vi "set_in_library.vi"(2 "Cluster":T4, 3 "camera cluster":T3, 4 "Tracker Handle":i32, 5 "Array":dbl[][](array[numeric])) -> (0 "No Error":bool, 1 "Directory Exists?":bool)   [LabVIEW 2010]
uses:
  <vilib>/vision/Avi1.llb/AviRefnum.ctl
  <vilib>/userDefined/High Color/IMAQdx.ctl
  lib/MWT.dll
panel:
  out "return type 9":i32
  out "return type 8":i32
  out "return type 7":i32
  out "return type 6":i32
  out "return type 5":i32
  out "return type 4":i32
  out "return type 3":i32
  out "return type 2":i32
  out "return type":i32
  in  "ObjectFrames of Persistence":i32=5
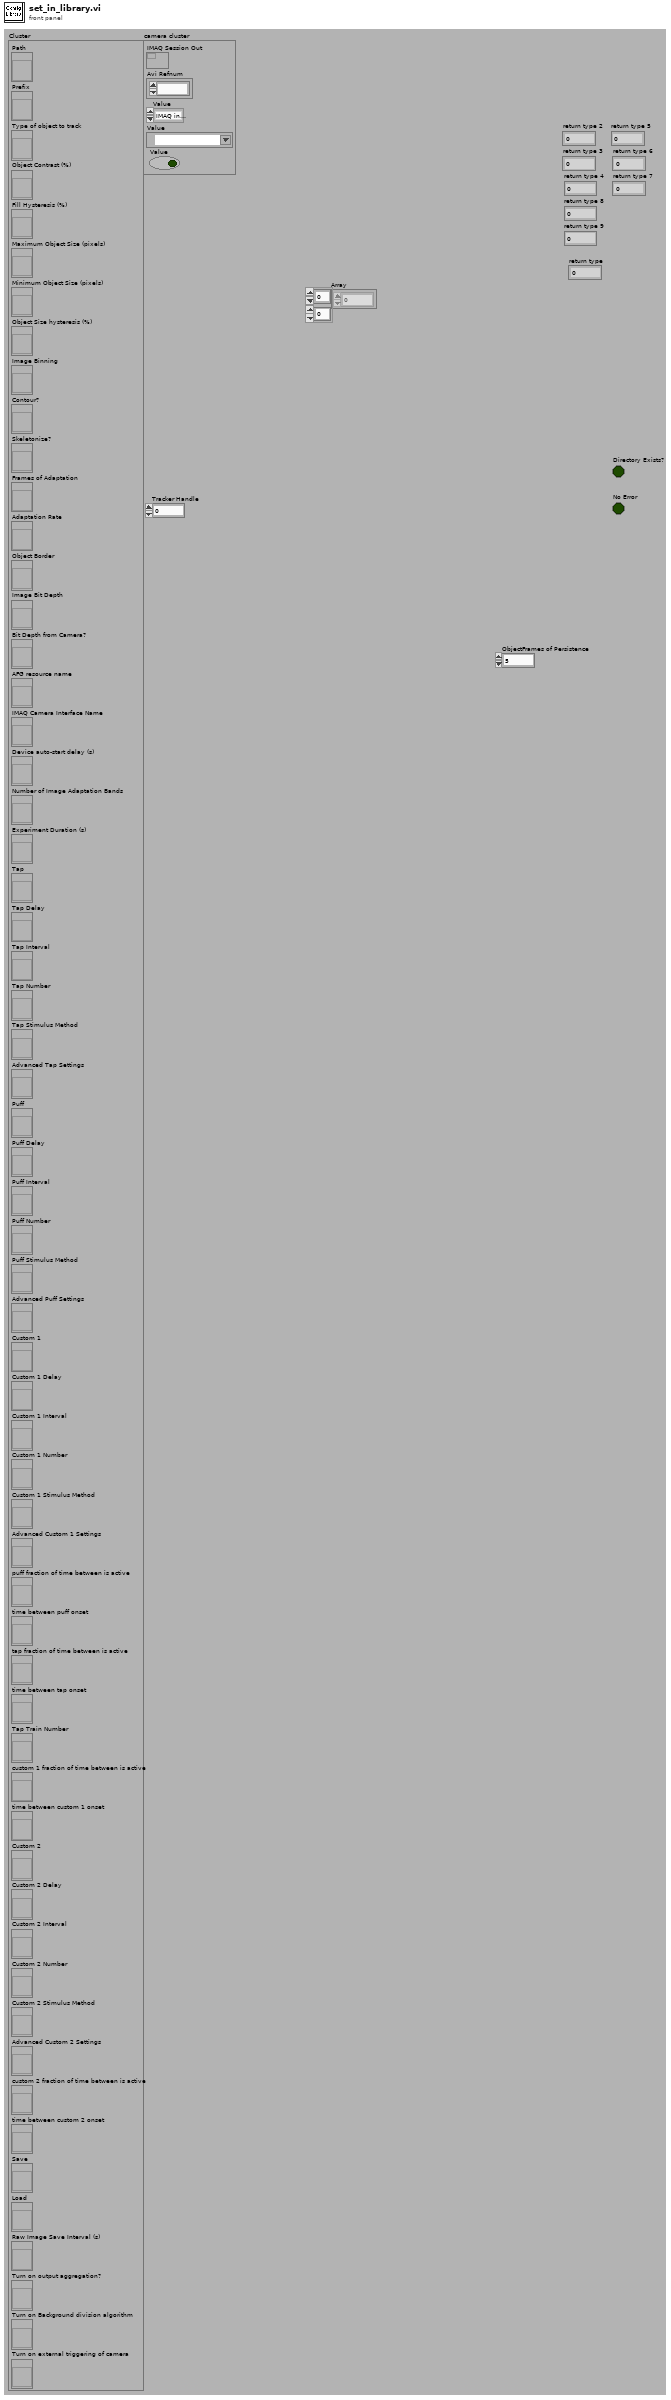
[diagram p1: front panel]
types:
  T1 = typedef "AviRefnum.ctl" = refnum<k1>
  T2 = typedef "IMAQdx.ctl" = refnum<k21>
  T3 = cluster{"IMAQ Session Out":refnum<k11>, "Avi Refnum":T1, "Value":enum32{"IMAQ interface", "IMAQdx interface", "AVI file"}, "Value":T2, "Value":bool}
  T4 = cluster{"Path":refnum<vi>, "Prefix":refnum<vi>, "Type of object to track":refnum<vi>, "Object Contrast (%)":refnum<vi>, "Fill Hysteresis (%)":refnum<vi>, "Maximum Object Size (pixels)":refnum<vi>, "Minimum Object Size (pixels)":refnum<vi>, "Object Size hysteresis (%)":refnum<vi>, "Image Binning":refnum<vi>, "Contour?":refnum<vi>, "Skeletonize?":refnum<vi>, "Frames of Adaptation":refnum<vi>, "Adaptation Rate":refnum<vi>, "Object Border":refnum<vi>, "Image Bit Depth":refnum<vi>, "Bit Depth from Camera?":refnum<vi>, "AFG resource name":refnum<vi>, "IMAQ Camera Interface Name":refnum<vi>, "Device auto-start delay (s)":refnum<vi>, "Number of Image Adaptation Bands":refnum<vi>, "Experiment Duration (s)":refnum<vi>, "Tap":refnum<vi>, "Tap Delay":refnum<vi>, "Tap Interval":refnum<vi>, "Tap Number":refnum<vi>, "Tap Stimulus Method":refnum<vi>, "Advanced Tap Settings":refnum<vi>, "Puff":refnum<vi>, "Puff Delay":refnum<vi>, "Puff Interval":refnum<vi>, "Puff Number":refnum<vi>, "Puff Stimulus Method":refnum<vi>, "Advanced Puff Settings":refnum<vi>, "Custom 1":refnum<vi>, "Custom 1 Delay":refnum<vi>, "Custom 1 Interval":refnum<vi>, "Custom 1 Number":refnum<vi>, "Custom 1 Stimulus Method":refnum<vi>, "Advanced Custom 1 Settings":refnum<vi>, "puff fraction of time between is active":refnum<vi>, "time between puff onset":refnum<vi>, "tap fraction of time between is active":refnum<vi>, "time between tap onset":refnum<vi>, "Tap Train Number":refnum<vi>, "custom 1 fraction of time between is active":refnum<vi>, "time between custom 1 onset":refnum<vi>, "Custom 2":refnum<vi>, "Custom 2 Delay":refnum<vi>, "Custom 2 Interval":refnum<vi>, "Custom 2 Number":refnum<vi>, "Custom 2 Stimulus Method":refnum<vi>, "Advanced Custom 2 Settings":refnum<vi>, "custom 2 fraction of time between is active":refnum<vi>, "time between custom 2 onset":refnum<vi>, "Save":refnum<vi>, "Load":refnum<vi>, "Raw Image Save Interval (s)":refnum<vi>, "Turn on output aggregation?":refnum<vi>, "Turn on Background division algorithm":refnum<vi>, "Turn on external triggering of camera":refnum<vi>}
  T5 = cluster{"Value":path, "Value":string, "Value":bool, "Value":dbl, "Value":dbl, "Value":i32, "Value":i32, "Value":dbl, "Value":u16, "Value":bool, "Value":bool, "Value":i32, "Value":i32, "Value":i32, "Value":u32, "Value":i32, "Value":bool}
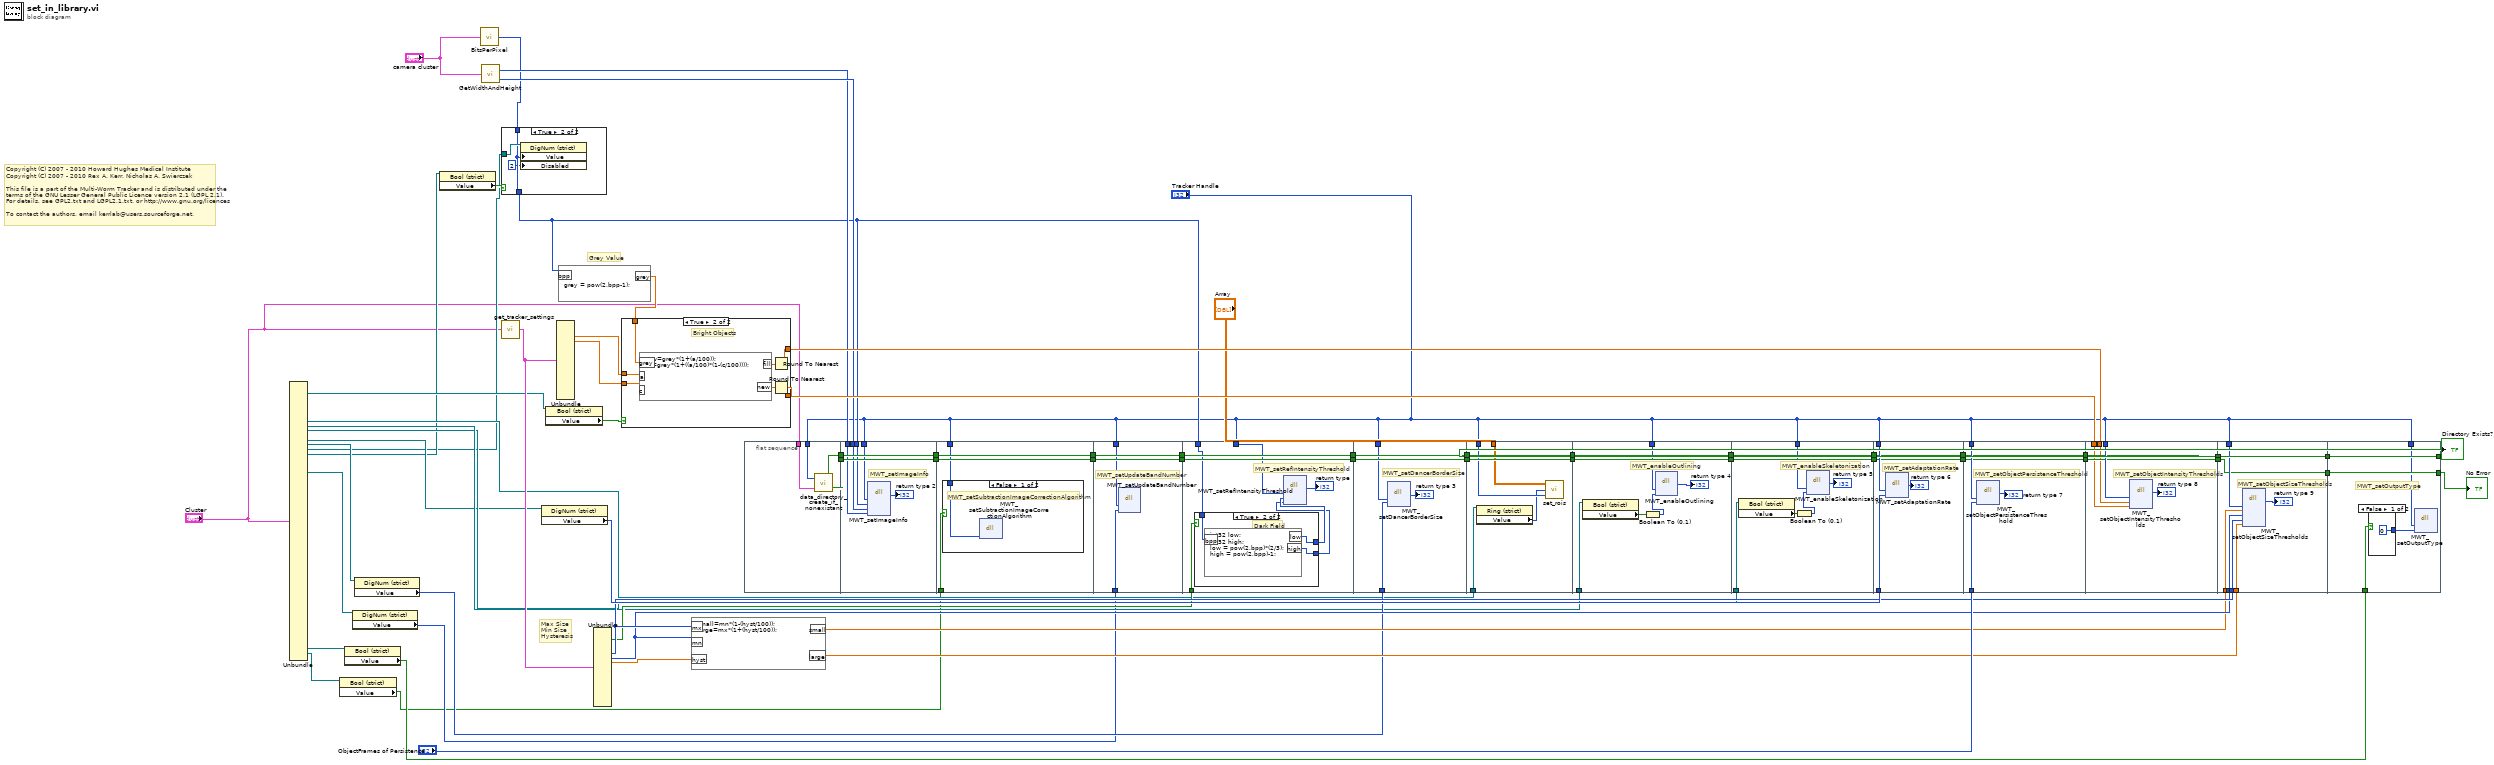
[diagram p0: block diagram]
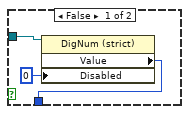
[diagram p2: hidden frame]
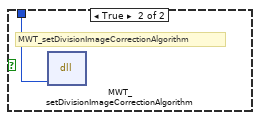
[diagram p3: hidden frame]
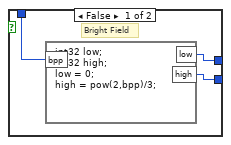
[diagram p4: hidden frame]
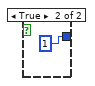
[diagram p5: hidden frame]
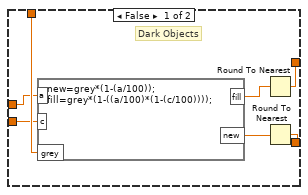
[diagram p6: hidden frame]
diagram:
  # "Copyright (C) 2007 - 2010 Howard Hughes Medical Institute\nCopyright (C) 2007 - 2010 Rex A. Kerr, Nicholas A. Swierczek\n \nThis file is a part of the Multi-Worm Tracker and is distributed under the\nterms of the GNU Lesser General Public Licence version 2.1 (LGPL 2.1).\nFor details, see GPL2.txt and LGPL2.1.txt, or http://www.gnu.org/licences\n \nTo contact the authors, email kerrlab@users.sourceforge.net."
  # "Max Size\nMin Size\nHysteresis"
  # "Grey Value"
  n1 = Unbundle("Cluster") -> ("Type of object to track"=w25:refnum<vi>, "Image Binning"=w24:refnum<vi>, "Contour?"=w23:refnum<vi>, "Skeletonize?"=w22:refnum<vi>, "Adaptation Rate"=w21:refnum<vi>, "Object Border"=w20:refnum<vi>, "Image Bit Depth"=w18:refnum<vi>, "Bit Depth from Camera?"=w19:refnum<vi>, "Number of Image Adaptation Bands"=w15:refnum<vi>, "Turn on output aggregation?"=w11:refnum<vi>, "Turn on Background division algorithm"=w5:refnum<vi>)  [unwired: 49 out]
  n2 = property class="Bool (strict)"(reference=w5) -> ("Value"=w4:bool)  [unwired: 1 in, 2 out]
  n3 = property class="Bool (strict)"(reference=w11) -> ("Value"=w10:bool)  [unwired: 1 in, 2 out]
  n4 = property class="DigNum (strict)"(reference=w15) -> ("Value"=w14:i32)  [unwired: 1 in, 2 out]
  n5 = property class="DigNum (strict)"(reference=w20) -> ("Value"=w31:i32)  [unwired: 1 in, 2 out]
  n6 = property class="Bool (strict)"(reference=w19) -> ("Value"=w42:bool)  [unwired: 1 in, 2 out]
  n7 = call "BitsPerPixel.vi"("camera cluster"="camera cluster") -> ("BitsPerPixel"=w28:u32)
  n8 = call "GetWidthAndHeight.vi"("camera cluster"="camera cluster") -> ("Width"=w29:u32, "Height"=w30:u32)
  n9 = call "get_tracker_settings.vi"("Cluster"="Cluster") -> ("settings value cluster"=w66:T5)
  n10 = case shown="True" w42 {
    tunnel: [w69 w72] -> w27
    tunnel: w28 -> [_ w72]
    tunnel: w18 -> [w70 w73]
    frame False {
      n11 = property class="DigNum (strict)"(reference=w70, "Disabled"=u8 0) -> ("Value"=w69:u32)  [unwired: 1 in, 2 out]
    }
    frame True {
      n12 = property class="DigNum (strict)"(reference=w73, "Value"=w72, "Disabled"=u8 2) -> ()  [unwired: 1 in, 2 out]
    }
  }
  n13 = property class="DigNum (strict)"(reference=w21) -> ("Value"=w62:i32)  [unwired: 1 in, 2 out]
  n14 = property class="Bool (strict)"(reference=w25) -> ("Value"=w67:bool)  [unwired: 1 in, 2 out]
  n15 = Unbundle(w66) -> ("Value"=w37:dbl, "Value"=w65:dbl)  [unwired: 15 out]
  n16 = formula code="grey = pow(2,bpp-1);"("bpp"=w27) -> ("grey"=w43:dbl)
  n17 = Unbundle(w66) -> ("Value"=w26:bool, "Value"=w36:i32, "Value"=w35:i32, "Value"=w34:dbl)  [unwired: 13 out]
  n18 = case shown="True" w67 {
    tunnel: w43 -> [w80 w87]
    tunnel: w37 -> [w79 w86]
    tunnel: w65 -> [w78 w85]
    tunnel: [w74 w81] -> w64
    tunnel: [w76 w83] -> w63
    frame False {
      # "Dark Objects"
      n19 = formula code="new=grey*(1-(a/100));\nfill=grey*(1-((a/100)*(1-(c/100))));"("a"=w79, "c"=w78, "grey"=w80) -> ("new"=w77:dbl, "fill"=w75:dbl)
      n20 = Round To Nearest(number=w75) -> (nearest integer value=w74:dbl)
      n21 = Round To Nearest(number=w77) -> (nearest integer value=w76:dbl)
    }
    frame True {
      # "Bright Objects"
      n22 = formula code="new=grey*(1+(a/100));\nfill=grey*(1+((a/100)*(1-(c/100))));"("a"=w86, "c"=w85, "grey"=w87) -> ("new"=w84:dbl, "fill"=w82:dbl)
      n23 = Round To Nearest(number=w82) -> (nearest integer value=w81:dbl)
      n24 = Round To Nearest(number=w84) -> (nearest integer value=w83:dbl)
    }
  }
  n25 = formula code="small=mn*(1-(hyst/100));\nlarge=mx*(1+(hyst/100));"("mx"=w36, "mn"=w35, "hyst"=w34) -> ("small"=w33:dbl, "large"=w32:dbl)
  n26 = flat-sequence {
    tunnel: [w91] -> w45
    tunnel: [w90] -> w44
    tunnel: "Tracker Handle" -> [w89]
    tunnel: "Cluster" -> [w88]
    tunnel: w45 -> [w98]
    tunnel: [w98] -> w9
    tunnel: w44 -> [w97]
    tunnel: [w97] -> w7
    tunnel: "Tracker Handle" -> [w96]
    tunnel: w27 -> [w95]
    tunnel: w29 -> [w94]
    tunnel: w30 -> [w93]
    tunnel: w9 -> [w102]
    tunnel: [w102] -> w8
    tunnel: w7 -> [w101]
    tunnel: [w101] -> w6
    tunnel: w4 -> [w100]
    tunnel: "Tracker Handle" -> [w99]
    tunnel: w8 -> [w108]
    tunnel: [w108] -> w17
    tunnel: w6 -> [w107]
    tunnel: [w107] -> w16
    tunnel: "Tracker Handle" -> [w106]
    tunnel: w14 -> [w105]
    tunnel: w17 -> [w116]
    tunnel: [w116] -> w49
    tunnel: w16 -> [w115]
    tunnel: [w115] -> w47
    tunnel: "Tracker Handle" -> [w114]
    tunnel: w27 -> [w111]
    tunnel: w26 -> [w112]
    tunnel: w49 -> [w127]
    tunnel: [w127] -> w48
    tunnel: w47 -> [w126]
    tunnel: [w126] -> w46
    tunnel: "Tracker Handle" -> [w125]
    tunnel: w31 -> [w124]
    tunnel: w48 -> [w133]
    tunnel: [w133] -> w41
    tunnel: w46 -> [w132]
    tunnel: [w132] -> w39
    tunnel: "Array" -> [w131]
    tunnel: "Tracker Handle" -> [w130]
    tunnel: w24 -> [w129]
    tunnel: w41 -> [w140]
    tunnel: [w140] -> w40
    tunnel: w39 -> [w139]
    tunnel: [w139] -> w38
    tunnel: "Tracker Handle" -> [w136]
    tunnel: w23 -> [w135]
    tunnel: [w147] -> w57
    tunnel: w40 -> [w147]
    tunnel: w38 -> [w146]
    tunnel: [w146] -> w56
    tunnel: "Tracker Handle" -> [w145]
    tunnel: w22 -> [w144]
    tunnel: w62 -> [w152]
    tunnel: "Tracker Handle" -> [w151]
    tunnel: [w150] -> w58
    tunnel: w57 -> [w150]
    tunnel: w56 -> [w149]
    tunnel: [w149] -> w55
    tunnel: "ObjectFrames of Persistence" -> [w157]
    tunnel: "Tracker Handle" -> [w156]
    tunnel: [w155] -> w59
    tunnel: w58 -> [w155]
    tunnel: w55 -> [w154]
    tunnel: [w154] -> w54
    tunnel: w64 -> [w159]
    tunnel: w63 -> [w160]
    tunnel: "Tracker Handle" -> [w163]
    tunnel: [w162] -> w60
    tunnel: w59 -> [w162]
    tunnel: w54 -> [w161]
    tunnel: [w161] -> w53
    tunnel: w33 -> [w171]
    tunnel: w35 -> [w170]
    tunnel: w36 -> [w169]
    tunnel: w32 -> [w168]
    tunnel: "Tracker Handle" -> [w167]
    tunnel: w60 -> [w166]
    tunnel: w53 -> [w165]
    tunnel: [w166] -> w13
    tunnel: [w165] -> w12
    tunnel: [w175] -> w51
    tunnel: [w176] -> w52
    tunnel: w13 -> [w176]
    tunnel: w12 -> [w175]
    tunnel: "Tracker Handle" -> [w173]
    tunnel: w10 -> [w172]
    frame #0 {
      n27 = call "data_directory_create_if_nonexistant.vi"("Cluster"=w88, "Tracker Handle"=w89) -> ("Error"=w90:bool, "Directory Exists?"=w91:bool)
    }
    frame #1 {
      # "MWT_setImageInfo"
      n28 = dll-call lib="C:/MWT/lib/MWT.dll" fn="MWT_setImageInfo"("handle"=w96, "bits"=w95, "width"=w93, "height"=w94) -> ("return type"=→"return type 2":i32)  [unwired: 7 in, 2 out]
    }
    frame #2 {
      n29 = case shown="False" w100 {
        tunnel: w99 -> [w103 w104]
        frame False {
          # "MWT_setSubtractionImageCorrectionAlgorithm"
          n30 = dll-call lib="C:/MWT/lib/MWT.dll" fn="MWT_setSubtractionImageCorrectionAlgorithm"("handle"=w103) -> ()  [unwired: 5 in, 2 out]
        }
        frame True {
          # "MWT_setDivisionImageCorrectionAlgorithm"
          n31 = dll-call lib="C:/MWT/lib/MWT.dll" fn="MWT_setDivisionImageCorrectionAlgorithm"("handle"=w104) -> ()  [unwired: 5 in, 2 out]
        }
      }
    }
    frame #3 {
      # "MWT_setUpdateBandNumber"
      n32 = dll-call lib="C:/MWT/lib/MWT.dll" fn="MWT_setUpdateBandNumber"("handle"=w106, "num_bands"=w105) -> ()  [unwired: 6 in, 2 out]
    }
    frame #4 {
      # "MWT_setRefIntensityThreshold"
      n33 = case shown="True" w112 {
        tunnel: [w119 w122] -> w110
        tunnel: [w118 w121] -> w109
        tunnel: w111 -> [w117 w120]
        frame False {
          # "Bright Field"
          n34 = formula code="int32 low;\nint32 high;\nlow = 0;\nhigh = pow(2,bpp)/3;"("bpp"=w117) -> ("low"=w119:i32, "high"=w118:i32)
        }
        frame True {
          # "Dark Field"
          n35 = formula code="int32 low;\nint32 high;\nlow = pow(2,bpp)*(2/3);\nhigh = pow(2,bpp)-1;"("bpp"=w120) -> ("low"=w122:i32, "high"=w121:i32)
        }
      }
      n36 = dll-call lib="C:/MWT/lib/MWT.dll" fn="MWT_setRefIntensityThreshold"("handle"=w114, "intensity_low"=w110, "intensity_high"=w109) -> ("return type"=→"return type":i32)  [unwired: 6 in, 2 out]
    }
    frame #5 {
      # "MWT_setDancerBorderSize"
      n37 = dll-call lib="C:/MWT/lib/MWT.dll" fn="MWT_setDancerBorderSize"("handle"=w125, "border_size"=w124) -> ("return type"=→"return type 3":i32)  [unwired: 5 in, 2 out]
    }
    frame #6 {
      n38 = property class="Ring (strict)"(reference=w129) -> ("Value"=w128:u16)  [unwired: 1 in, 2 out]
      n39 = call "set_rois.vi"("Tracker Handle"=w130, "Binning"=w128, "Array"=w131) -> ()
    }
    frame #7 {
      # "MWT_enableOutlining"
      n40 = property class="Bool (strict)"(reference=w135) -> ("Value"=w137:bool)  [unwired: 1 in, 2 out]
      n41 = Boolean To (0,1)(Boolean=w137) -> (0, 1=w138:i16)
      n42 = dll-call lib="C:/MWT/lib/MWT.dll" fn="MWT_enableOutlining"("handle"=w136, "enable"=w138) -> ("return type"=→"return type 4":i32)  [unwired: 5 in, 2 out]
    }
    frame #8 {
      # "MWT_enableSkeletonization"
      n43 = property class="Bool (strict)"(reference=w144) -> ("Value"=w143:bool)  [unwired: 1 in, 2 out]
      n44 = Boolean To (0,1)(Boolean=w143) -> (0, 1=w142:i16)
      n45 = dll-call lib="C:/MWT/lib/MWT.dll" fn="MWT_enableSkeletonization"("handle"=w145, "enable"=w142) -> ("return type"=→"return type 5":i32)  [unwired: 5 in, 2 out]
    }
    frame #9 {
      # "MWT_setAdaptationRate"
      n46 = dll-call lib="C:/MWT/lib/MWT.dll" fn="MWT_setAdaptationRate"("handle"=w151, "alpha"=w152) -> ("return type"=→"return type 6":i32)  [unwired: 5 in, 2 out]
    }
    frame #10 {
      # "MWT_setObjectPersistenceThreshold"
      n47 = dll-call lib="C:/MWT/lib/MWT.dll" fn="MWT_setObjectPersistenceThreshold"("handle"=w156, "frames_of_persistence"=w157) -> ("return type"=→"return type 7":i32)  [unwired: 5 in, 2 out]
    }
    frame #11 {
      # "MWT_setObjectIntensityThresholds"
      n48 = dll-call lib="C:/MWT/lib/MWT.dll" fn="MWT_setObjectIntensityThresholds"("handle"=w163, "intensity_to_fill"=w159, "intensity_of_new"=w160) -> ("return type"=→"return type 8":i32)  [unwired: 6 in, 2 out]
    }
    frame #12 {
      # "MWT_setObjectSizeThresholds"
      n49 = dll-call lib="C:/MWT/lib/MWT.dll" fn="MWT_setObjectSizeThresholds"("handle"=w167, "small_size"=w171, "small_good_size"=w170, "large_good_size"=w169, "large_size"=w168) -> ("return type"=→"return type 9":i32)  [unwired: 8 in, 2 out]
    }
    frame #13 {
      # "MWT_setOutputType"
      n50 = case shown="False" w172 {
        tunnel: [0 1] -> w174
        frame False {
        }
        frame True {
        }
      }
      n51 = dll-call lib="C:/MWT/lib/MWT.dll" fn="MWT_setOutputType"("handle"=w173, "type"=w174) -> ()  [unwired: 6 in, 2 out]
    }
  }
  "Directory Exists?" <- w52
  "No Error" <- w51
